vi "Send Open Actor Core FP.vi"(7 "Message Priority (Normal)":T1=enum."Normal", 8 "error in (no error)":errorcluster, 10 "Open FP (F)":bool, 11 "Message Enqueuer":refnum<class "Message Enqueuer.lvclass">) -> (0 "error out":errorcluster, 3 "Message Enqueuer out":refnum<class "Message Enqueuer.lvclass">)   [LabVIEW 2015, in "CS++BaseActor.lvlib" / "Open Actor Core FP Msg.lvclass"]
doc: "Sends the <B>CS++BaseActor.lvlib:Open Actor Core FP Msg.lvclass</B> message.\n\n<B>CS++BaseActor.lvlib:CS++BaseActor.lvclass:Open Actor Core FP.vi</B> Description:\n\nOpen or close <b>Actor Core.vi</B> frontpanel."
uses:
  Open Actor Core FP Msg.lvclass
  <vilib>/ActorFramework/Message Enqueuer/Message Enqueuer.lvclass
  <vilib>/ActorFramework/Message Enqueuer/Message Priority.ctl
  Open Actor Core FP Msg.lvclass/Open Actor Core FP Msg.ctl
  <vilib>/ActorFramework/Message Enqueuer/Message Enqueuer.lvclass/Message Enqueuer.ctl
  <vilib>/ActorFramework/Message Priority Queue/Priority Enqueue.vi
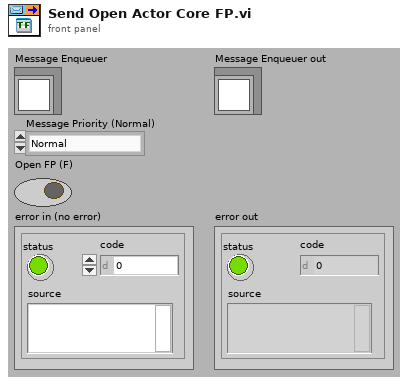
[diagram p1: front panel]
types:
  T1 = typedef "Actor Framework.lvlib/Message Enqueuer.lvclass/Message Priority.ctl" = enum16{"Low", "Normal", "High"}
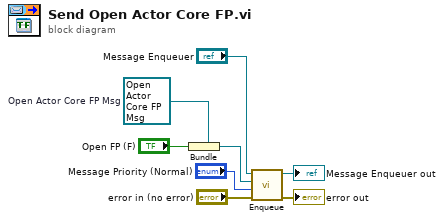
[diagram p0: block diagram]
diagram:
  w2 = refnum<class "Open Actor Core FP Msg.lvclass"> refnum  # Open Actor Core FP Msg
  n1 = Bundle(cluster=w2, "Open FP (F)") -> (w5:refnum<class "Open Actor Core FP Msg.lvclass">)
  n2 = call <vilib>:"Enqueue.vi"("error in (no error)"="error in (no error)", "Message Priority (Normal)"="Message Priority (Normal)", "Message"=w5, "Message Enqueuer in"="Message Enqueuer") -> ("error out"=→"error out":errorcluster, "Message Enqueuer out"=→"Message Enqueuer out":refnum<class "Message Enqueuer.lvclass">)  [unwired: 6 in]
